vi "Inficon 16 Bit Data.vi"(8 "error in (no error)":errorcluster, 10 "Emerson Flow Meter Data Input":T1, 11 "Modbus Master in":refnum<class "Modbus Master.lvclass">=refnum) -> (0 "error out":errorcluster, 2 "Emerson Flow Meter Data Output":T1={"Gross Heating Value, Vol (Real, Dry)"=65535.0, "Nitrogen Component Normalized Mole % (Dry)"=8.0, "Methane Component Normalized Mole % (Dry)"=69.0, "Carbon Dioxide Component Normalized Mole % (Dry)"=65535.0, "Ethane Component Normalized Mole % (Dry)"=65.0, "Propane Component Normalized Mole % (Dry)"=8.0, "i-Pentane Component Normalized Mole % (Dry)"=14.0, "i-Butane Component Normalized Mole % (Dry)"=66.0, "n-Butane Component Normalized Mole % (Dry)"=8.0, "n-Pentane Component Normalized Mole % (Dry)"=0.0, "Hexane Component Normalized Mole % (Dry)"=0.0, "Heptane Component Normalized Mole % (Dry)"=0.0, "Gross Wobbe Index, Real(Dry)"=0.0, "Relative Density, Real(Dry)"=40.0, "Propylene Component Normalized Mole % (Dry)"=0.0, "C4 Olefins Component Normalized Mole % (Dry)"=0.0, "Water Component Normalized Mole % (Dry)"=0.0}, 3 "Modbus Master out":refnum<class "Modbus Master.lvclass">)   [LabVIEW 2019]
uses:
  <vilib>/NI/Modbus Library/API/Master/Modbus Master.lvclass
  Type Definitions/Inficon Modbus Addresses.ctl
  Type Definitions/Inficon Data.ctl
  <vilib>/NI/Modbus Library/Transmission Data Unit/IP/IP Data Unit.lvclass
  <vilib>/NI/Modbus Library/Master Function Definition/Master Function Definition.lvclass
  <vilib>/NI/Modbus Library/Network Protocol/Network Master/TCP/TCP Master.lvclass
panel:
  in  "CMD 17":T2=46 items=["Gross Heating Value (Dry)"=100, "Nitrogen"=102, "Methane"=104, "CO2"=106, "Ethane"=108, "Propane"=110, "i-Butane"=112, "n-Butane"=114, "i-Pentane"=116, "n-Pentane"=118, "Hexane"=120, "Heptane"=122, "Gross Wobbe Index (Dry)"=124, "Relative Density (Dry)"=126]
  in  "CMD 16":T2=45 items=["Gross Heating Value (Dry)"=100, "Nitrogen"=102, "Methane"=104, "CO2"=106, "Ethane"=108, "Propane"=110, "i-Butane"=112, "n-Butane"=114, "i-Pentane"=116, "n-Pentane"=118, "Hexane"=120, "Heptane"=122, "Gross Wobbe Index (Dry)"=124, "Relative Density (Dry)"=126]
  in  "CMD 15":T2=44 items=["Gross Heating Value (Dry)"=100, "Nitrogen"=102, "Methane"=104, "CO2"=106, "Ethane"=108, "Propane"=110, "i-Butane"=112, "n-Butane"=114, "i-Pentane"=116, "n-Pentane"=118, "Hexane"=120, "Heptane"=122, "Gross Wobbe Index (Dry)"=124, "Relative Density (Dry)"=126]
  in  "CMD 14":T2=42 items=["Gross Heating Value (Dry)"=100, "Nitrogen"=102, "Methane"=104, "CO2"=106, "Ethane"=108, "Propane"=110, "i-Butane"=112, "n-Butane"=114, "i-Pentane"=116, "n-Pentane"=118, "Hexane"=120, "Heptane"=122, "Gross Wobbe Index (Dry)"=124, "Relative Density (Dry)"=126]
  in  "CMD 13":T2=41 items=["Gross Heating Value (Dry)"=100, "Nitrogen"=102, "Methane"=104, "CO2"=106, "Ethane"=108, "Propane"=110, "i-Butane"=112, "n-Butane"=114, "i-Pentane"=116, "n-Pentane"=118, "Hexane"=120, "Heptane"=122, "Gross Wobbe Index (Dry)"=124, "Relative Density (Dry)"=126]
  in  "CMD 12":T2=40 items=["Gross Heating Value (Dry)"=100, "Nitrogen"=102, "Methane"=104, "CO2"=106, "Ethane"=108, "Propane"=110, "i-Butane"=112, "n-Butane"=114, "i-Pentane"=116, "n-Pentane"=118, "Hexane"=120, "Heptane"=122, "Gross Wobbe Index (Dry)"=124, "Relative Density (Dry)"=126]
  in  "CMD 11":T2=39 items=["Gross Heating Value (Dry)"=100, "Nitrogen"=102, "Methane"=104, "CO2"=106, "Ethane"=108, "Propane"=110, "i-Butane"=112, "n-Butane"=114, "i-Pentane"=116, "n-Pentane"=118, "Hexane"=120, "Heptane"=122, "Gross Wobbe Index (Dry)"=124, "Relative Density (Dry)"=126]
  in  "CMD 10":T2=17 items=["Gross Heating Value (Dry)"=100, "Nitrogen"=102, "Methane"=104, "CO2"=106, "Ethane"=108, "Propane"=110, "i-Butane"=112, "n-Butane"=114, "i-Pentane"=116, "n-Pentane"=118, "Hexane"=120, "Heptane"=122, "Gross Wobbe Index (Dry)"=124, "Relative Density (Dry)"=126]
  in  "CMD 9":T2=16 items=["Gross Heating Value (Dry)"=100, "Nitrogen"=102, "Methane"=104, "CO2"=106, "Ethane"=108, "Propane"=110, "i-Butane"=112, "n-Butane"=114, "i-Pentane"=116, "n-Pentane"=118, "Hexane"=120, "Heptane"=122, "Gross Wobbe Index (Dry)"=124, "Relative Density (Dry)"=126]
  in  "CMD 8":T2=11 items=["Gross Heating Value (Dry)"=100, "Nitrogen"=102, "Methane"=104, "CO2"=106, "Ethane"=108, "Propane"=110, "i-Butane"=112, "n-Butane"=114, "i-Pentane"=116, "n-Pentane"=118, "Hexane"=120, "Heptane"=122, "Gross Wobbe Index (Dry)"=124, "Relative Density (Dry)"=126]
  in  "CMD 7":T2=10 items=["Gross Heating Value (Dry)"=100, "Nitrogen"=102, "Methane"=104, "CO2"=106, "Ethane"=108, "Propane"=110, "i-Butane"=112, "n-Butane"=114, "i-Pentane"=116, "n-Pentane"=118, "Hexane"=120, "Heptane"=122, "Gross Wobbe Index (Dry)"=124, "Relative Density (Dry)"=126]
  in  "CMD 6":T2=9 items=["Gross Heating Value (Dry)"=100, "Nitrogen"=102, "Methane"=104, "CO2"=106, "Ethane"=108, "Propane"=110, "i-Butane"=112, "n-Butane"=114, "i-Pentane"=116, "n-Pentane"=118, "Hexane"=120, "Heptane"=122, "Gross Wobbe Index (Dry)"=124, "Relative Density (Dry)"=126]
  in  "CMD 5":T2=8 items=["Gross Heating Value (Dry)"=100, "Nitrogen"=102, "Methane"=104, "CO2"=106, "Ethane"=108, "Propane"=110, "i-Butane"=112, "n-Butane"=114, "i-Pentane"=116, "n-Pentane"=118, "Hexane"=120, "Heptane"=122, "Gross Wobbe Index (Dry)"=124, "Relative Density (Dry)"=126]
  in  "CMD 4":T2=5 items=["Gross Heating Value (Dry)"=100, "Nitrogen"=102, "Methane"=104, "CO2"=106, "Ethane"=108, "Propane"=110, "i-Butane"=112, "n-Butane"=114, "i-Pentane"=116, "n-Pentane"=118, "Hexane"=120, "Heptane"=122, "Gross Wobbe Index (Dry)"=124, "Relative Density (Dry)"=126]
  in  "CMD 3":T2=4 items=["Gross Heating Value (Dry)"=100, "Nitrogen"=102, "Methane"=104, "CO2"=106, "Ethane"=108, "Propane"=110, "i-Butane"=112, "n-Butane"=114, "i-Pentane"=116, "n-Pentane"=118, "Hexane"=120, "Heptane"=122, "Gross Wobbe Index (Dry)"=124, "Relative Density (Dry)"=126]
  in  "CMD 2":T2=3 items=["Gross Heating Value (Dry)"=100, "Nitrogen"=102, "Methane"=104, "CO2"=106, "Ethane"=108, "Propane"=110, "i-Butane"=112, "n-Butane"=114, "i-Pentane"=116, "n-Pentane"=118, "Hexane"=120, "Heptane"=122, "Gross Wobbe Index (Dry)"=124, "Relative Density (Dry)"=126]
  in  "CMD 1":T2=2 items=["Gross Heating Value (Dry)"=100, "Nitrogen"=102, "Methane"=104, "CO2"=106, "Ethane"=108, "Propane"=110, "i-Butane"=112, "n-Butane"=114, "i-Pentane"=116, "n-Pentane"=118, "Hexane"=120, "Heptane"=122, "Gross Wobbe Index (Dry)"=124, "Relative Density (Dry)"=126]
  # "Natural Gas"
  # "Propane"
  # "Natural Gas"
  # "Propane"
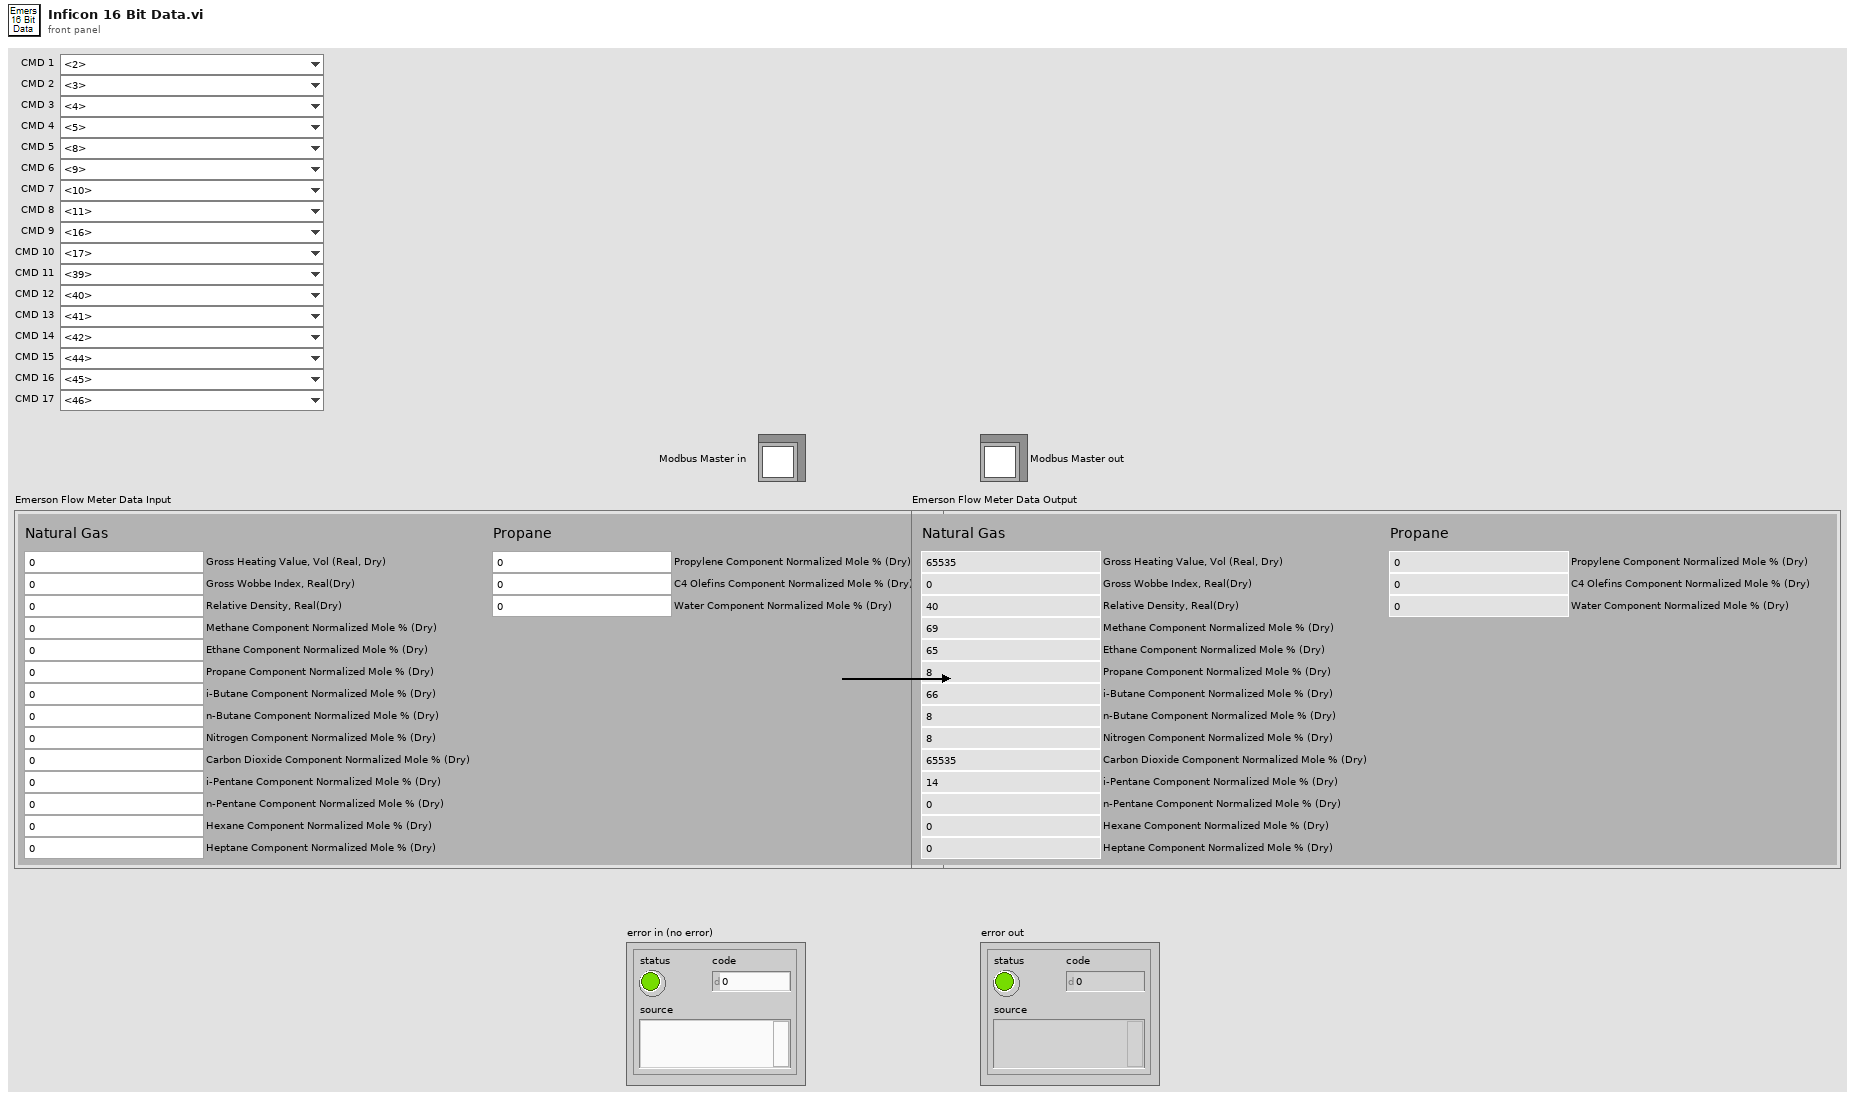
[diagram p1: front panel]
types:
  T1 = typedef "Inficon Data.ctl" = cluster{"Gross Heating Value, Vol (Real, Dry)":dbl, "Nitrogen Component Normalized Mole % (Dry)":dbl, "Methane Component Normalized Mole % (Dry)":dbl, "Carbon Dioxide Component Normalized Mole % (Dry)":dbl, "Ethane Component Normalized Mole % (Dry)":dbl, "Propane Component Normalized Mole % (Dry)":dbl, "i-Pentane Component Normalized Mole % (Dry)":dbl, "i-Butane Component Normalized Mole % (Dry)":dbl, "n-Butane Component Normalized Mole % (Dry)":dbl, "n-Pentane Component Normalized Mole % (Dry)":dbl, "Hexane Component Normalized Mole % (Dry)":dbl, "Heptane Component Normalized Mole % (Dry)":dbl, "Gross Wobbe Index, Real(Dry)":dbl, "Relative Density, Real(Dry)":dbl, "Propylene Component Normalized Mole % (Dry)":dbl, "C4 Olefins Component Normalized Mole % (Dry)":dbl, "Water Component Normalized Mole % (Dry)":dbl}
  T2 = typedef "Inficon Modbus Addresses.ctl" = u16
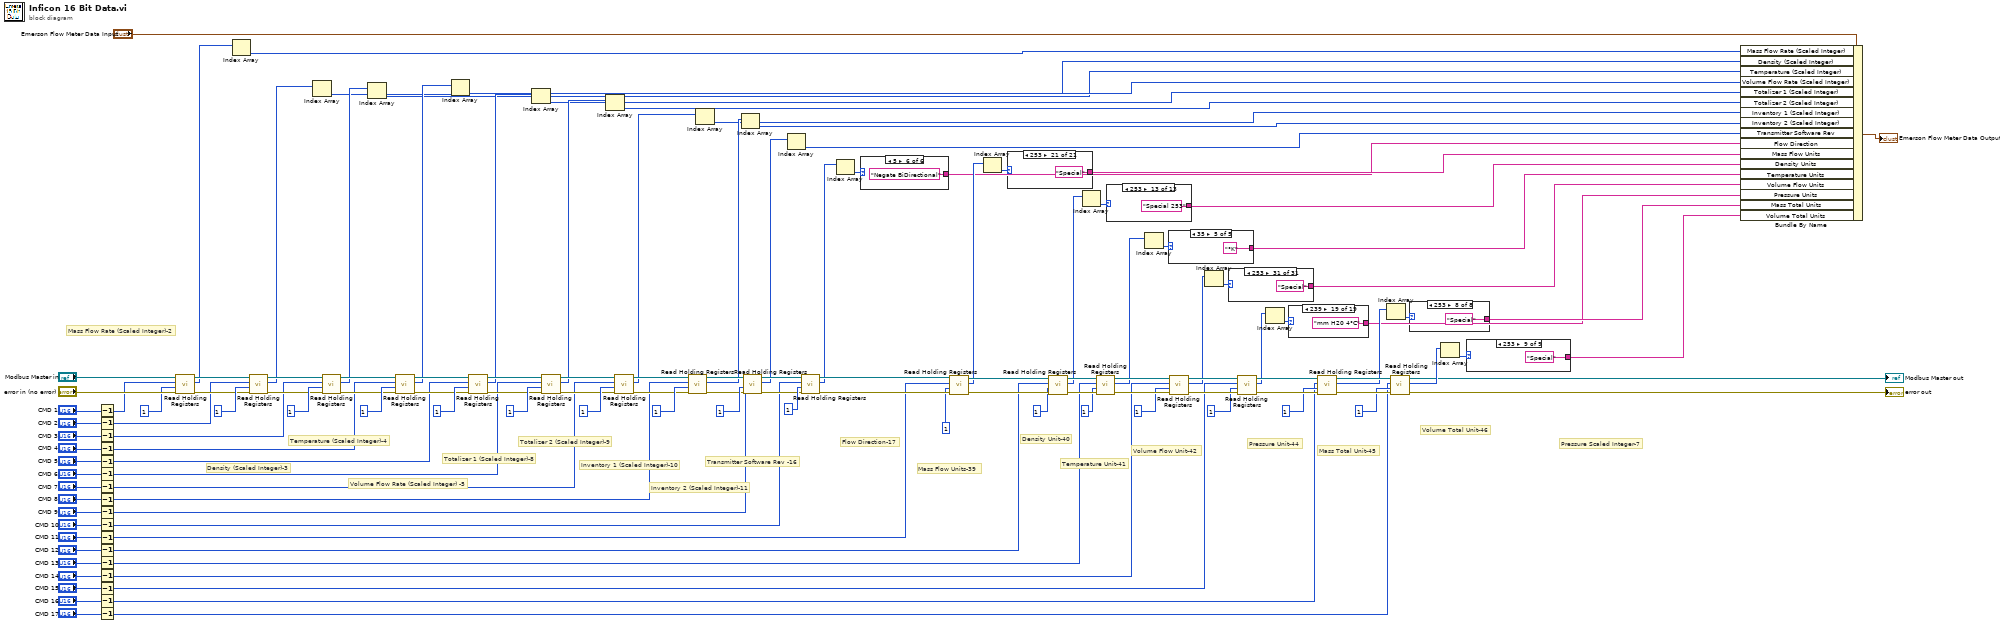
[diagram p0: block diagram]
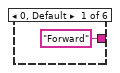
[diagram p2: hidden frame]
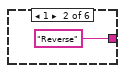
[diagram p3: hidden frame]
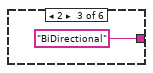
[diagram p4: hidden frame]
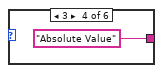
[diagram p5: hidden frame]
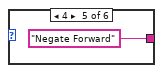
[diagram p6: hidden frame]
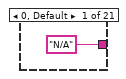
[diagram p7: hidden frame]
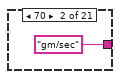
[diagram p8: hidden frame]
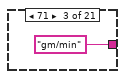
[diagram p9: hidden frame]
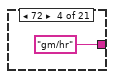
[diagram p10: hidden frame]
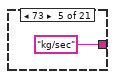
[diagram p11: hidden frame]
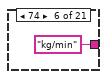
[diagram p12: hidden frame]
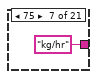
[diagram p13: hidden frame]
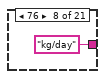
[diagram p14: hidden frame]
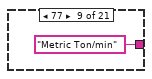
[diagram p15: hidden frame]
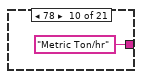
[diagram p16: hidden frame]
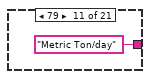
[diagram p17: hidden frame]
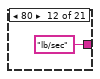
[diagram p18: hidden frame]
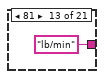
[diagram p19: hidden frame]
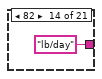
[diagram p20: hidden frame]
diagram:
  # "Pressure Scaled Integer-7"
  # "Volume Total Unit-46"
  # "Mass Total Unit-45"
  # "Pressure Unit-44"
  # "Volume Flow Unit-42"
  # "Temperature Unit-41"
  # "Density Unit-40"
  # "Mass Flow Units-39"
  # "Flow Direction-17"
  # "Transmitter Software Rev -16"
  # "Inventory 2 (Scaled Integer)-11"
  # "Inventory 1 (Scaled Integer)-10"
  # "Totalizer 2 (Scaled Integer)-9"
  # "Totalizer 1 (Scaled Integer)-8"
  # "Volume Flow Rate (Scaled Integer) -5"
  # "Temperature (Scaled Integer)-4"
  # "Density (Scaled Integer)-3"
  # "Mass Flow Rate (Scaled Integer)-2"
  n1 = Decrement(x="CMD 1") -> (x-1=w77:T2)
  n2 = Decrement(x="CMD 2") -> (x-1=w75:T2)
  n3 = Decrement(x="CMD 3") -> (x-1=w73:T2)
  n4 = Decrement(x="CMD 4") -> (x-1=w71:T2)
  n5 = Decrement(x="CMD 5") -> (x-1=w69:T2)
  n6 = Decrement(x="CMD 6") -> (x-1=w67:T2)
  n7 = Decrement(x="CMD 7") -> (x-1=w65:T2)
  n8 = Decrement(x="CMD 8") -> (x-1=w63:T2)
  n9 = Decrement(x="CMD 9") -> (x-1=w61:T2)
  n10 = Decrement(x="CMD 10") -> (x-1=w59:T2)
  n11 = Decrement(x="CMD 11") -> (x-1=w57:T2)
  n12 = Decrement(x="CMD 12") -> (x-1=w55:T2)
  n13 = Decrement(x="CMD 13") -> (x-1=w53:T2)
  n14 = Decrement(x="CMD 14") -> (x-1=w51:T2)
  n15 = Decrement(x="CMD 15") -> (x-1=w49:T2)
  n16 = Decrement(x="CMD 16") -> (x-1=w47:T2)
  n17 = Decrement(x="CMD 17") -> (x-1=w45:T2)
  n18 = call-dynamic "Read Holding Registers.vi"("error in"="error in (no error)", "number of inputs"=u16 1, "starting address"=w77, "Modbus master in"="Modbus Master in") -> ("error out"=w100:errorcluster, "register values"=w4:u16[], "Modbus master out"=w101:refnum<class "Modbus Master.lvclass">)  [unwired: 5 in]
  n19 = Index Array(array=w4) -> (element=w3:u16)  [unwired: 1 in]
  n20 = call-dynamic "Read Holding Registers.vi"("error in"=w100, "number of inputs"=u16 1, "starting address"=w75, "Modbus master in"=w101) -> ("error out"=w98:errorcluster, "register values"=w6:u16[], "Modbus master out"=w97:refnum<class "Modbus Master.lvclass">)  [unwired: 5 in]
  n21 = Index Array(array=w6) -> (element=w5:u16)  [unwired: 1 in]
  n22 = call-dynamic "Read Holding Registers.vi"("error in"=w98, "number of inputs"=u16 1, "starting address"=w73, "Modbus master in"=w97) -> ("error out"=w95:errorcluster, "register values"=w8:u16[], "Modbus master out"=w94:refnum<class "Modbus Master.lvclass">)  [unwired: 5 in]
  n23 = Index Array(array=w8) -> (element=w7:u16)  [unwired: 1 in]
  n24 = call-dynamic "Read Holding Registers.vi"("error in"=w95, "number of inputs"=u16 1, "starting address"=w71, "Modbus master in"=w94) -> ("error out"=w92:errorcluster, "register values"=w10:u16[], "Modbus master out"=w91:refnum<class "Modbus Master.lvclass">)  [unwired: 5 in]
  n25 = Index Array(array=w10) -> (element=w9:u16)  [unwired: 1 in]
  n26 = call-dynamic "Read Holding Registers.vi"("error in"=w92, "number of inputs"=u16 1, "starting address"=w69, "Modbus master in"=w91) -> ("error out"=w89:errorcluster, "register values"=w12:u16[], "Modbus master out"=w88:refnum<class "Modbus Master.lvclass">)  [unwired: 5 in]
  n27 = Index Array(array=w12) -> (element=w11:u16)  [unwired: 1 in]
  n28 = call-dynamic "Read Holding Registers.vi"("error in"=w89, "number of inputs"=u16 1, "starting address"=w67, "Modbus master in"=w88) -> ("error out"=w86:errorcluster, "register values"=w14:u16[], "Modbus master out"=w85:refnum<class "Modbus Master.lvclass">)  [unwired: 5 in]
  n29 = Index Array(array=w14) -> (element=w13:u16)  [unwired: 1 in]
  n30 = call-dynamic "Read Holding Registers.vi"("error in"=w86, "number of inputs"=u16 1, "starting address"=w65, "Modbus master in"=w85) -> ("error out"=w83:errorcluster, "register values"=w16:u16[], "Modbus master out"=w82:refnum<class "Modbus Master.lvclass">)  [unwired: 5 in]
  n31 = call-dynamic "Read Holding Registers.vi"("error in"=w83, "number of inputs"=u16 1, "starting address"=w63, "Modbus master in"=w82) -> ("error out"=w80:errorcluster, "register values"=w18:u16[], "Modbus master out"=w79:refnum<class "Modbus Master.lvclass">)  [unwired: 5 in]
  n32 = Index Array(array=w16) -> (element=w15:u16)  [unwired: 1 in]
  n33 = Index Array(array=w18) -> (element=w17:u16)  [unwired: 1 in]
  n34 = call-dynamic "Read Holding Registers.vi"("error in"=w80, "number of inputs"=u16 1, "starting address"=w61, "Modbus master in"=w79) -> ("error out"=w128:errorcluster, "register values"=w20:u16[], "Modbus master out"=w127:refnum<class "Modbus Master.lvclass">)  [unwired: 5 in]
  n35 = Index Array(array=w20) -> (element=w19:u16)  [unwired: 1 in]
  n36 = call-dynamic "Read Holding Registers.vi"("error in"=w128, "number of inputs"=u16 1, "starting address"=w59, "Modbus master in"=w127) -> ("error out"=w126:errorcluster, "register values"=w22:u16[], "Modbus master out"=w119:refnum<class "Modbus Master.lvclass">)  [unwired: 5 in]
  n37 = Index Array(array=w22) -> (element=w23:u16)  [unwired: 1 in]
  n38 = case shown="5" w23 {
    tunnel: ["Forward" "Reverse" "BiDirectional" "Absolute Value" "Negate Forward" "Negate BiDirectional"] -> w21
    frame 0, Default {
    }
    frame 1 {
    }
    frame 2 {
    }
    frame 3 {
    }
    frame 4 {
    }
    frame 5 {
    }
  }
  n39 = call-dynamic "Read Holding Registers.vi"("error in"=w126, "number of inputs"=u16 1, "starting address"=w57, "Modbus master in"=w119) -> ("error out"=w125:errorcluster, "register values"=w25:u16[], "Modbus master out"=w118:refnum<class "Modbus Master.lvclass">)  [unwired: 5 in]
  n40 = Index Array(array=w25) -> (element=w26:u16)  [unwired: 1 in]
  n41 = case shown="253" w26 {
    tunnel: ["N/A" "gm/sec" "gm/min" "gm/hr" "kg/sec" "kg/min" "kg/hr" "kg/day" "Metric Ton/min" "Metric Ton/hr" "Metric Ton/day" "lb/sec" "lb/min" "lb/day" "lb/day" "Short Ton/min" "Short Ton/hr" "Short Ton/day" "Long Ton/hr" "Long Ton/day" "Special"] -> w24
    frame 0, Default {
    }
    frame 70 {
    }
    frame 71 {
    }
    frame 72 {
    }
    frame 73 {
    }
    frame 74 {
    }
    frame 75 {
    }
    frame 76 {
    }
    frame 77 {
    }
    frame 78 {
    }
    frame 79 {
    }
    frame 80 {
    }
    frame 81 {
    }
    frame 82 {
    }
    frame 83 {
    }
    frame 84 {
    }
    frame 85 {
    }
    frame 86 {
    }
    frame 87 {
    }
    frame 88 {
    }
    frame 253 {
    }
  }
  n42 = call-dynamic "Read Holding Registers.vi"("error in"=w125, "number of inputs"=u16 1, "starting address"=w55, "Modbus master in"=w118) -> ("error out"=w124:errorcluster, "register values"=w28:u16[], "Modbus master out"=w117:refnum<class "Modbus Master.lvclass">)  [unwired: 5 in]
  n43 = Index Array(array=w28) -> (element=w29:u16)  [unwired: 1 in]
  n44 = call-dynamic "Read Holding Registers.vi"("error in"=w124, "number of inputs"=u16 1, "starting address"=w53, "Modbus master in"=w117) -> ("error out"=w123:errorcluster, "register values"=w31:u16[], "Modbus master out"=w116:refnum<class "Modbus Master.lvclass">)  [unwired: 5 in]
  n45 = case shown="253" w29 {
    tunnel: ["N/A" "Specific Gravity" "gm/cm³" "kg/m³" "lb/US Gal" "lb/ft³" "gm/mL" "kg/L" "gm/L" "lb/in³" "Short Ton/yd³" "Degrees_API" "Special 253"] -> w27
    frame 0, Default {
    }
    frame 90 {
    }
    frame 91 {
    }
    frame 92 {
    }
    frame 93 {
    }
    frame 94 {
    }
    frame 95 {
    }
    frame 96 {
    }
    frame 97 {
    }
    frame 98 {
    }
    frame 99 {
    }
    frame 104 {
    }
    frame 253 {
    }
  }
  n46 = Index Array(array=w31) -> (element=w32:u16)  [unwired: 1 in]
  n47 = case shown="35" w32 {
    tunnel: ["N/A" "°C" "°F" "°R" "°K"] -> w30
    frame 0, Default {
    }
    frame 32 {
    }
    frame 33 {
    }
    frame 34 {
    }
    frame 35 {
    }
  }
  n48 = call-dynamic "Read Holding Registers.vi"("error in"=w123, "number of inputs"=u16 1, "starting address"=w51, "Modbus master in"=w116) -> ("error out"=w122:errorcluster, "register values"=w34:u16[], "Modbus master out"=w115:refnum<class "Modbus Master.lvclass">)  [unwired: 5 in]
  n49 = Index Array(array=w34) -> (element=w35:u16)  [unwired: 1 in]
  n50 = case shown="253" w35 {
    tunnel: ["N/A" "ft³/min" "US GPM" "LPM" "IMP GPM" "m³/hr" "US Gal/Sec" "Million US Gal/Day" "L/s" "Million L/day" "ft³/s" "ft³/day" "m³/sec" "m³/day" "Imp Gal/hr" "Imp Gal/day" "ft³/hr" "m³/min" "Barrels/sec" "Barrels/min" "Barrels/hr" "Barrels/day" "US Gal/hr" "Imp Gal/sec" "L/hr" "Barrels/sec" "Barrels/min" "Barrels/hour" "Barrels/day" "US Gal/day" "Special"] -> w33
    frame 0, Default {
    }
    frame 15 {
    }
    frame 16 {
    }
    frame 17 {
    }
    frame 18 {
    }
    frame 19 {
    }
    frame 22 {
    }
    frame 23 {
    }
    frame 24 {
    }
    frame 25 {
    }
    frame 26 {
    }
    frame 27 {
    }
    frame 28 {
    }
    frame 29 {
    }
    frame 30 {
    }
    frame 31 {
    }
    frame 130 {
    }
    frame 131 {
    }
    frame 132 {
    }
    frame 133 {
    }
    frame 134 {
    }
    frame 135 {
    }
    frame 136 {
    }
    frame 137 {
    }
    frame 138 {
    }
    frame 170 {
    }
    frame 171 {
    }
    frame 172 {
    }
    frame 173 {
    }
    frame 235 {
    }
    frame 253 {
    }
  }
  n51 = call-dynamic "Read Holding Registers.vi"("error in"=w122, "number of inputs"=u16 1, "starting address"=w49, "Modbus master in"=w115) -> ("error out"=w121:errorcluster, "register values"=w37:u16[], "Modbus master out"=w114:refnum<class "Modbus Master.lvclass">)  [unwired: 5 in]
  n52 = Index Array(array=w37) -> (element=w38:u16)  [unwired: 1 in]
  n53 = case shown="239" w38 {
    tunnel: ["N/A" "in H20 68°F" "IN HG 0°C" "Ft H20 68°F" "mm H20 68°F" "mm HG 0°C" "PSI" "BAR" "mBAR" "gm/cm²" "kg/cm²" "Pa" "kPa" "Torr 0°C" "atm" "IN H20 60°F" "MPa" "IN H20 4°C" "mm H20 4°C"] -> w36
    frame 0, Default {
    }
    frame 1 {
    }
    frame 2 {
    }
    frame 3 {
    }
    frame 4 {
    }
    frame 5 {
    }
    frame 6 {
    }
    frame 7 {
    }
    frame 8 {
    }
    frame 9 {
    }
    frame 10 {
    }
    frame 11 {
    }
    frame 12 {
    }
    frame 13 {
    }
    frame 14 {
    }
    frame 145 {
    }
    frame 237 {
    }
    frame 238 {
    }
    frame 239 {
    }
  }
  n54 = call-dynamic "Read Holding Registers.vi"("error in"=w121, "number of inputs"=u16 1, "starting address"=w47, "Modbus master in"=w114) -> ("error out"=w120:errorcluster, "register values"=w40:u16[], "Modbus master out"=w113:refnum<class "Modbus Master.lvclass">)  [unwired: 5 in]
  n55 = Index Array(array=w40) -> (element=w41:u16)  [unwired: 1 in]
  n56 = call-dynamic "Read Holding Registers.vi"("error in"=w120, "number of inputs"=u16 1, "starting address"=w45, "Modbus master in"=w113) -> ("error out"=→"error out":errorcluster, "register values"=w44:u16[], "Modbus master out"=→"Modbus Master out":refnum<class "Modbus Master.lvclass">)  [unwired: 5 in]
  n57 = case shown="253" w41 {
    tunnel: ["N/A" "Grams" "Kilograms" "Metric Tons" "lbs" "Short Ton 2000lb" "Long Ton 2240lb" "Special"] -> w39
    frame 0, Default {
    }
    frame 60 {
    }
    frame 61 {
    }
    frame 62 {
    }
    frame 63 {
    }
    frame 64 {
    }
    frame 65 {
    }
    frame 253 {
    }
  }
  n58 = Index Array(array=w44) -> (element=w43:u16)  [unwired: 1 in]
  n59 = case shown="253" w43 {
    tunnel: ["N/A" "US Gallon" "Liters" "Imperial Gallons" "m³" "Barrels (42 US Gallons)" "ft³" "Beer Barrels" "Special"] -> w42
    frame 0, Default {
    }
    frame 40 {
    }
    frame 41 {
    }
    frame 42 {
    }
    frame 43 {
    }
    frame 46 {
    }
    frame 112 {
    }
    frame 170 {
    }
    frame 253 {
    }
  }
  n60 = Bundle By Name(cluster="Emerson Flow Meter Data Input", "Mass Flow Rate (Scaled Integer)"=w3, "Density (Scaled Integer)"=w5, "Temperature (Scaled Integer)"=w7, "Volume Flow Rate (Scaled Integer)"=w9, "Totalizer 1 (Scaled Integer)"=w11, "Totalizer 2 (Scaled Integer)"=w13, "Inventory 1 (Scaled Integer)"=w15, "Inventory 2 (Scaled Integer)"=w17, "Transmitter Software Rev"=w19, "Flow Direction"=w21, "Mass Flow Units"=w24, "Density Units"=w27, "Temperature Units"=w30, "Volume Flow Units"=w33, "Pressure Units"=w36, "Mass Total Units"=w39, "Volume Total Units"=w42) -> (→"Emerson Flow Meter Data Output":T1)
